vi "GetGasIndex.vi"(7 "Timeout (ms)":u32=2000, 8 "Error In":errorcluster, 11 "Sierra M100 In":refnum<visa-resource-name>) -> (0 "Error Out":errorcluster, 2 "Gas Index":u16, 3 "Sierra M100 Out":refnum<visa-resource-name>)   [LabVIEW 2012, in "Sierra-M100.lvlib"]
doc: "This VI gets the gas index for the mass flow controller. The gas index is an indicator of the calibration gas. Use \"Get Gas\" VI instead."
uses:
  Sierra-M100.lvlib
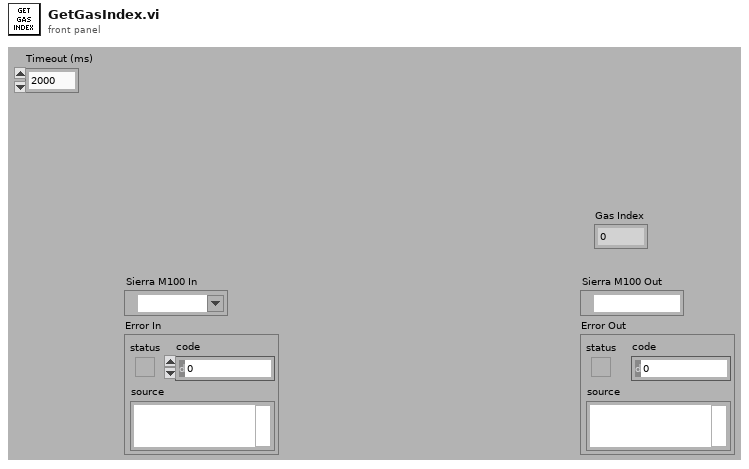
[diagram p1: front panel]
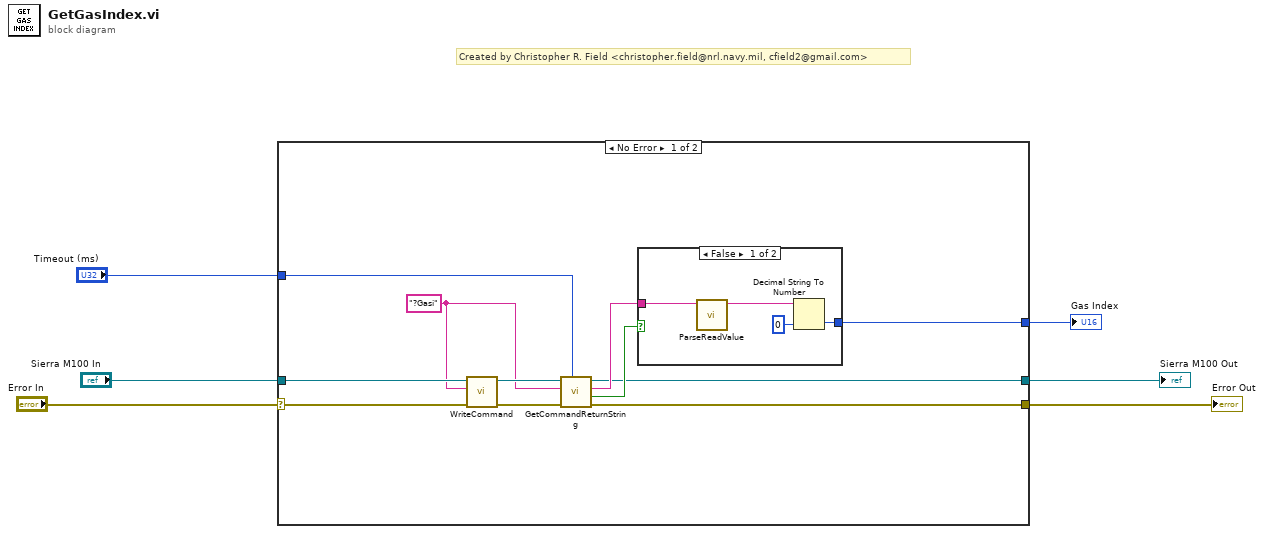
[diagram p0: block diagram]
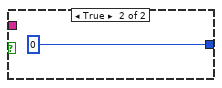
[diagram p2: hidden frame]
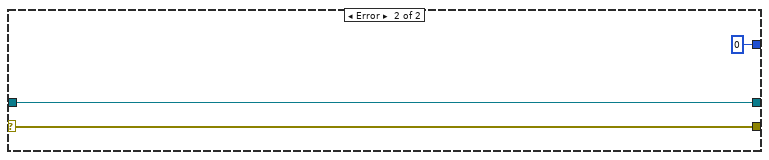
[diagram p3: hidden frame]
diagram:
  # "Created by Christopher R. Field <christopher.field@nrl.navy.mil, cfield2@gmail.com>"
  n1 = case shown="No Error" "Error In" {
    selector: "Error In" -> [w7 w25]
    tunnel: "Sierra M100 In" -> [w17 w24]
    tunnel: [w16 u16 0] -> w5
    tunnel: "Timeout (ms)" -> [w12 _]
    tunnel: [w9 w24] -> w3
    tunnel: [w8 w25] -> w2
    frame No Error {
      w13 = "?Gasi"
      n2 = call "WriteCommand.vi"("Error In"=w7, "Command"=w13, "Sierra M100 In"=w17) -> ("Error Out"=w14:errorcluster, "Sierra M100 Out"=w15:refnum<visa-resource-name>)  [unwired: 5 in, 2 out]
      n3 = call "GetCommandReturnString.vi"("Timeout (ms)"=w12, "Error In"=w14, "Command"=w13, "Sierra M100 In"=w15) -> ("Error Out"=w8:errorcluster, "Timeout?"=w11:bool, "Return String"=w10:string, "Sierra M100 Out"=w9:refnum<visa-resource-name>)  [unwired: 4 in]
      n4 = case shown="False" w11 {
        tunnel: [w20 u16 0] -> w16
        tunnel: w10 -> [w19 _]
        frame False {
          n5 = call "ParseReadValue.vi"("Read Buffer"=w19) -> ("Value"=w18:string)  [unwired: 10 in]
          n6 = Decimal String To Number(string=w18, default (0L)=u16 0 ("default (0 I32)")) -> (number=w20:u16)  [unwired: 1 in, 1 out]
        }
        frame True {
        }
      }
    }
    frame Error {
    }
  }
  "Sierra M100 Out" <- w3
  "Error Out" <- w2
  "Gas Index" <- w5
